vi "Get Routes.vi"(4 "Promise in":refnum<class "Promise.lvclass">, 8 "error in (no error)":errorcluster, 11 "MuxActor in":refnum<class "MuxActor.lvclass">) -> (0 "error out":errorcluster, 3 "MuxActor out":refnum<class "MuxActor.lvclass">)   [LabVIEW 2022 SP3, in "VideoMux.lvlib" / "MuxActor.lvclass"]
uses:
  MuxActor.lvclass
  MuxActor.lvclass/MuxActor.ctl
  Mux/Mux.lvclass
  <vilib>/IlluminatedG/IG Promises/Promises/Promise/Promise.lvclass
  MuxRoute Value/MuxRoute Value.lvclass
  C:/Program Files (x86)/National Instruments/LabVIEW 2022/vi.lib/IlluminatedG/IG Promises/Promises/Value/Value.lvclass
  C:/dev/illuminatedg/TouchControl/VideoMux/MuxRoute Value/MuxRoute Value.lvclass
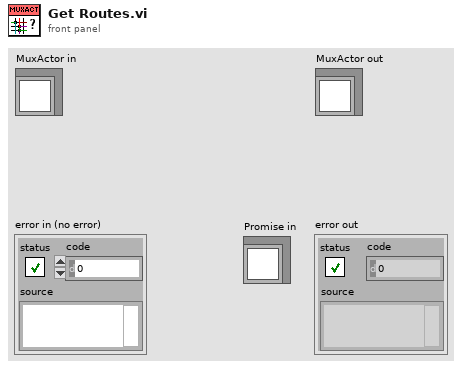
[diagram p1: front panel]
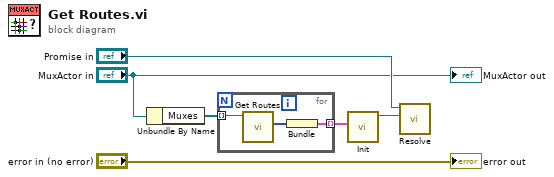
[diagram p0: block diagram]
diagram:
  n1 = Unbundle By Name("MuxActor in") -> ("Muxes"=w2:refnum<class "Mux.lvclass">[])
  n2 = for {
    tunnel: w2 -> [w9] mode=indexing
    tunnel: [w7] -> w5 mode=indexing
    n3 = call "Get Routes.vi"("Mux in"=w9) -> ("Routes"=w8:i32[])  [unwired: 8 in, 2 out]
    n4 = Bundle("Routes"=w8) -> (w7:cluster{"Routes":i32[]})  [unwired: 1 in]
  }
  n5 = call "Init.vi"("Muxes"=w5) -> ("MuxRoute Value out"=w4:refnum<class "MuxRoute Value.lvclass">)  [unwired: 9 in, 1 out]
  n6 = call <vilib>:"Resolve.vi"("Result"=w4, "Promise in"="Promise in") -> ()  [unwired: 8 in, 2 out]
  "error out" <- "error in (no error)"
  "MuxActor out" <- "MuxActor in"
